vi "Do you hear what i hear.vi"(11 "Path":path) -> (0 "Stop":bool, 2 "Time Elapsed":u32 format="%<%H:%M>t", 3 "Current Data":waveform(dbl)[](graph))   [LabVIEW 2015]
uses:
  <vilib>/sound2/lvsound2.llb/Sampling Mode.ctl
  <vilib>/sound2/lvsound2.llb/Sound File Info (path).vi
  <vilib>/sound2/lvsound2.llb/Sound File Read Open.vi
  <vilib>/sound2/lvsound2.llb/Sound File Read (DBL).vi
  <vilib>/sound2/lvsound2.llb/Sound Output Write (DBL).vi
panel:
  in  "Number of Samples/Iteration":i32=2500
  in  "Device ID":u32
  in  "Stop":bool
  out "Current Iteration":i32
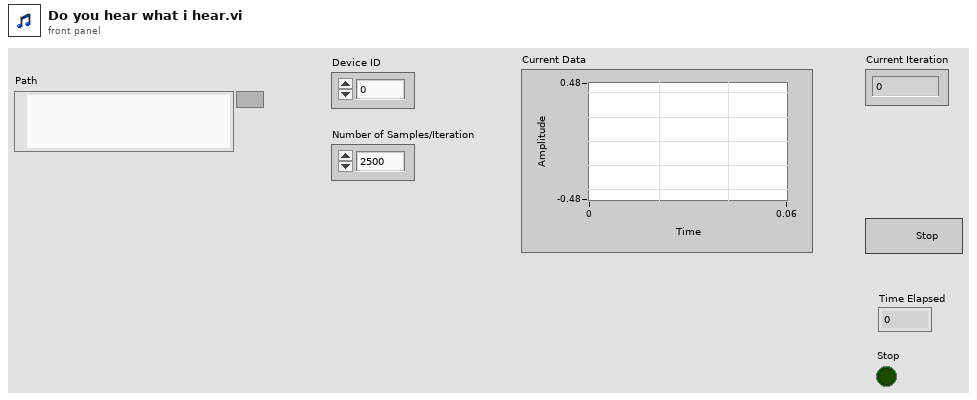
[diagram p1: front panel]
types:
  T1 = typedef "Sampling Mode.ctl" = i32
  T2 = typedef "Sound Data Format.ctl" = cluster{"sample rate (S/s)":dbl, "number of channels":i32, "bits per sample":i32}
  T3 = typedef "Sound File Refnum.ctl" = refnum<file>
  T4 = typedef "Sound Output Task ID.ctl" = u32
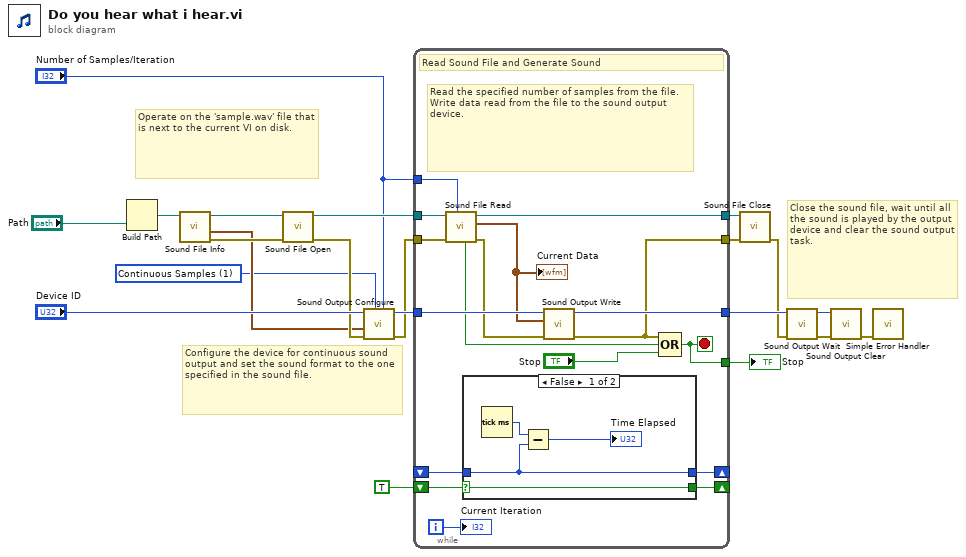
[diagram p0: block diagram]
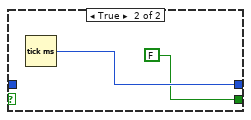
[diagram p2: hidden frame]
diagram:
  w6 = T1 1 items=["Finite Samples", "Continuous Samples"] ("sample mode")
  # "Operate on the 'sample.wav' file that is next to the current VI on disk."
  # "Close the sound file, wait until all the sound is played by the output device and clear the sound output task."
  # "Configure the device for continuous sound output and set the sound format to the one specified in the sound file."
  n1 = Build Path(name or relative path="Path") -> (appended path=w4:path)  [unwired: 1 in]
  n2 = call-poly <vilib>:"Sound File Info.vi"("path"=w4) -> ("error out"=w16:errorcluster, "sound format"=w8:T2, "path out"=w9:path)  [unwired: 7 in, 1 out]
  n3 = call-poly <vilib>:"Sound File Open.vi"("error in (no error)"=w16, "path"=w9) -> ("error out"=w15:errorcluster, "sound file refnum"=w17:T3)  [unwired: 8 in]
  n4 = call <vilib>:"Sound Output Configure.vi"("number of samples/ch"="Number of Samples/Iteration", "sample mode"=w6, "error in (no error)"=w15, "sound format"=w8, "device ID"="Device ID") -> ("error out"=w14:errorcluster, "task ID"=w21:T4)  [unwired: 5 in]
  n5 = while {
    tunnel: "Number of Samples/Iteration" -> [w29]
    tunnel: w17 -> [w36]
    tunnel: [w34] -> w19
    tunnel: w14 -> [w37]
    tunnel: [w28] -> w18
    tunnel: w21 -> [w33]
    tunnel: [w38] -> w12
    shift-right: [w26] -> _
    shift-left: _ -> [w25]
    shift-right: [w23] -> _
    shift-left: TRUE -> [w24]
    tunnel: [w22] -> w2
    i -> [w35]
    stop <- w22 stop-if-true
    # "Read the specified number of samples from the file. Write data read from the file to the sound output device."
    # "Read Sound File and Generate Sound"
    n6 = call-poly <vilib>:"Sound File Read.vi"("number of samples/ch (-1: all)"=w29, "error in (no error)"=w37, "sound file refnum"=w36) -> ("error out"=w32:errorcluster, "data"=w27:waveform(dbl)[], "sound file refnum out"=w34:T3, "end of file?"=w30:bool)  [unwired: 4 in, 1 out]
    "Current Data" <- w27
    n7 = case shown="False" w24 {
      selector: w24 -> [w42 _]
      tunnel: [w40 w44] -> w26
      tunnel: w25 -> [w40 _]
      tunnel: [w42 FALSE] -> w23
      frame False {
        n8 = Tick Count (ms)() -> (millisecond timer value=w41:u32)
        n9 = Subtract(x=w41, y=w40) -> (x-y=→"Time Elapsed":u32)
      }
      frame True {
        n10 = Tick Count (ms)() -> (millisecond timer value=w44:u32)
      }
    }
    n11 = call-poly <vilib>:"Sound Output Write.vi"("error in (no error)"=w32, "data"=w27, "task ID"=w33) -> ("error out"=w28:errorcluster, "task ID out"=w38:T4)  [unwired: 7 in]
    n12 = Compound Arithmetic op=OR(w28, w30, "Stop") -> (w22:bool)
    "Current Iteration" <- w35
  }
  "Stop" <- w2
  n13 = call <vilib>:"Sound File Close.vi"("error in (no error)"=w18, "sound file refnum"=w19) -> ("error out"=w11:errorcluster)  [unwired: 9 in]
  n14 = call <vilib>:"Sound Output Wait.vi"("error in (no error)"=w11, "task ID"=w12) -> ("error out"=w10:errorcluster, "task ID out"=w13:T4)  [unwired: 8 in]
  n15 = call <vilib>:"Sound Output Clear.vi"("error in (no error)"=w10, "task ID"=w13) -> ("error out"=w5:errorcluster)  [unwired: 9 in]
  n16 = call <vilib>:"Simple Error Handler.vi"("error in (no error)"=w5) -> ()  [unwired: 4 in, 5 out]
